vi "DataFinder_StorageVIs.vi"() -> ()   [LabVIEW 2023]
doc: "This example searches for channels in TDM files and TDMS files. The example uses the VIs \"Create Query\" and \"Execute Query\" to create and execute queries. The example then uses the \"Storage\" VIs to load the mass data of the found channels and graphically displays the data."
uses:
  <vilib>/DataFinder/DataTypes/object type.ctl
  <vilib>/DataFinder/DataTypes/comparison operator.ctl
  <vilib>/userdefined/High Color/DFDataFinder.ctl
  <vilib>/Platform/storage/lvStorage.llb/_openFunction.ctl
  <vilib>/DataFinder/Create Query (String).vi
  <vilib>/Platform/storage/lvStorage.llb/_openStorageWithRootAutoDetect.vi
  <vilib>/Platform/storage/lvStorage.llb/xStorage/xStorageSupp/ErrorOut.vi
  <vilib>/Platform/storage/lvStorage.llb/_queryPropPoly.vi
  <vilib>/Platform/storage/lvStorage.llb/_queryPropString.vi
  <vilib>/Platform/storage/lvStorage.llb/_queryGenericObjects.vi
  <vilib>/Platform/storage/lvStorage.llb/_loadAllDdt.vi
  <vilib>/Platform/storage/Storage.llb/Get Object Info.vi
  <vilib>/Platform/storage/Storage.llb/__closeStorageFromObject.vi
  <vilib>/DataFinder/Close Reference (Query).vi
  <vilib>/DataFinder/Close Reference (DataFinder).vi
  <vilib>/Platform/storage/lvStorage.llb/xStorage/Open Data Storage/Open Data Storage.xnode
  <vilib>/Platform/storage/lvStorage.llb/xStorage/Read Data/Read Data.xnode
  <vilib>/Platform/storage/lvStorage.llb/xStorage/Close Data Storage/Close Data Storage.xnode
  <vilib>/DataFinder/NI_DataFinder.lvlib
  <vilib>/userdefined/NI_DataFinder Controls.lvlib
panel:
  in  "DataFinder":T1
  in  "Operator":T2 items=["=", "<>", ">", "<", ">=", "<=", "#"]
  out "Result Signals":dynamicdata(graph)
  in  "Object Type":T3=2 items=["File", "Channel Group", "Channel"]
  in  "Value":string="Temp_A"
  in  "Property Name":string="name"
  out "Results Count":i32 min=0 max=0
  # "Overview: Executes a query for channels and uses the \"Storage\" VIs to display the mass data of the resulting channels.\nRequirements: Select a registered DataFinder which has indexed the TDM Server Demo Data.\nInstructions:\n1. Ensure that the selected DataFinder is already running.\n2. Specify a Query.\nTo use the predefined search values ensure the folder [all users]\\Documents\\National Instruments\\DataFinder or one of its parent folders is included in your search areas.\n3. Run the VI.\n4. View the Resulting Signals."
  # "Query"
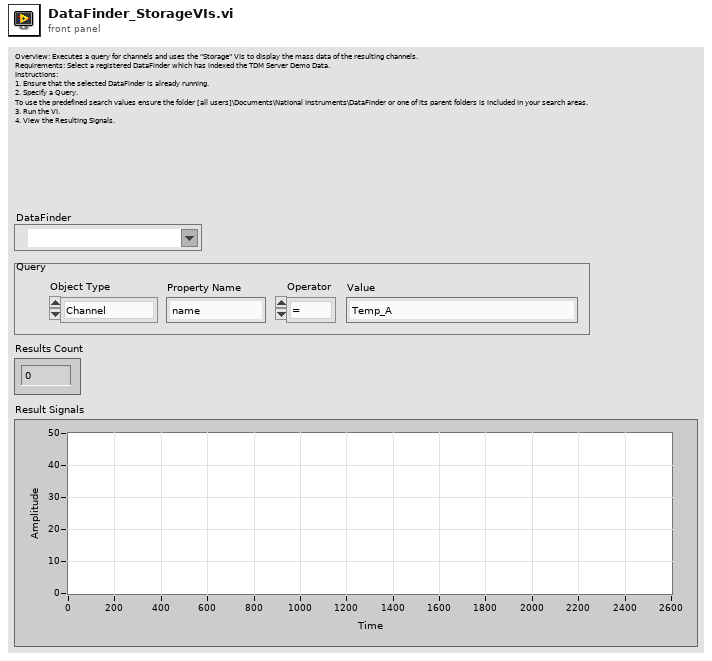
[diagram p1: front panel]
types:
  T1 = typedef "NI_DataFinder Controls.lvlib/DFDataFinder.ctl" = refnum<k21>
  T2 = typedef "NI_DataFinder.lvlib/comparison operator.ctl" = u16
  T3 = typedef "NI_DataFinder.lvlib/object type.ctl" = u16
  T4 = typedef "NI_DataFinder Controls.lvlib/DFQuery.ctl" = refnum<k20>
  T5 = typedef "NI_DataFinder.lvlib/results elements.ctl" = cluster{"fullpaths":path[], "DataPlugin names":string[], "channel group names":string[], "channel names":string[]}
  T6 = enum16{"UPDATE", "READ", "QUERY", "CREATE CHILD", "CREATE", "CONNECT", "DISCONNECT"}
  T7 = typedef "_openFunction.ctl" = enum16{"open", "open or create", "create or replace", "create", "open (read only)"}
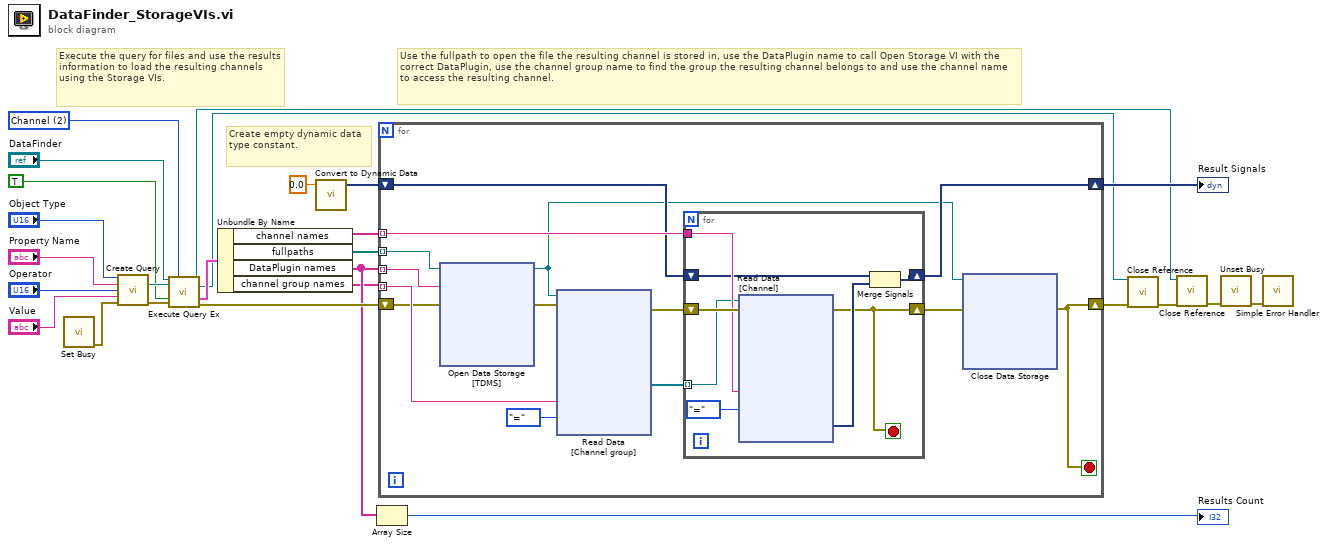
[diagram p0: block diagram]
diagram:
  w16 = T3 2 items=["File", "Channel Group", "Channel"] ("result object type (file)")
  # "Create empty dynamic data type constant."
  # "Use the fullpath to open the file the resulting channel is stored in, use the DataPlugin name to call Open Storage VI with the correct DataPlugin, use the channel group name to find the group the resulting channel belongs to and use the channel name to access the resulting channel."
  # "Execute the query for files and use the results information to load the resulting channels using the Storage VIs."
  n1 = call <vilib>:"Set Busy.vi"() -> ("error out"=w5:errorcluster)  [unwired: 10 in, 1 out]
  n2 = call-poly <vilib>:"Create Query.vi"("object type"="Object Type", "property name"="Property Name", "comparison operator (=)"="Operator", "value"="Value", "error in (no error)"=w5) -> ("query reference out"=w23:T4, "error out"=w24:errorcluster)  [unwired: 9 in]
  n3 = call <vilib>:"Execute Query Ex.vi"("DataFinder reference"="DataFinder", "result object type (file)"=w16, "query reference"=w23, "fill results elements? (F)"=TRUE, "error in (no error)"=w24) -> ("DataFinder reference out"=w9:T1, "query reference out"=w6:T4, "results elements"=w17:T5, "error out"=w18:errorcluster)  [unwired: 5 in, 2 out]
  n4 = Unbundle By Name(w17) -> ("channel names"=w12:string[], "fullpaths"=w13:path[], "DataPlugin names"=w15:string[], "channel group names"=w14:string[])
  n5 = call "Convert to Dynamic Data"("Double"=0.0) -> ("Dynamic Data Type"=w19:dynamicdata)  [unwired: 3 out]
  n6 = Array Size(array=w15) -> (size(s)=→"Results Count":i32)
  n7 = for {
    shift-right: [w33] -> w22
    shift-left: w19 -> [w34]
    shift-right: [w32] -> w8
    shift-left: w18 -> [w27]
    tunnel: w14 -> [w36] mode=indexing
    tunnel: w15 -> [w30] mode=indexing
    tunnel: w13 -> [w31] mode=indexing
    tunnel: w12 -> [w37] mode=indexing
    stop <- w32 stop-if-true
    n8 = xnode "Open Data Storage\n[TDMS]"("file path"=w31, "DataPlugin name"=w30, "error in (no error)"=w27) -> ("storage refnum (file)"=w28:refnum<k20>, "error out"=w29:errorcluster)  [unwired: 1 in, 2 out]
    n9 = xnode "Read Data\n[Channel group]"("Name"=w36, "Comparison (=)"=enum16{"=", "!=", ">", "<", ">=", "<="}."=", "storage refnum (file)"=w28, "error in"=w29) -> ("storage refnums (channel group)"=w35:refnum<k20>[], "error out"=w38:errorcluster)  [unwired: 1 out]
    n10 = for {
      tunnel: w37 -> [w71]
      shift-right: [w67] -> w33
      shift-left: w34 -> [w69]
      shift-right: [w65] -> w40
      shift-left: w38 -> [w72]
      tunnel: w35 -> [w66] mode=indexing
      stop <- w65 stop-if-true
      n11 = xnode "Read Data\n[Channel]"("Name"=w71, "Comparison (=)"=enum16{"=", "!=", ">", "<", ">=", "<="}."=", "storage refnum (channel group)"=w66, "error in"=w72) -> ("Signal"=w68:dynamicdata, "error out"=w65:errorcluster)  [unwired: 2 out]
      n12 = Merge Signals(w69, w68) -> (w67:dynamicdata)
    }
    n13 = xnode "Close Data Storage\n"("storage refnum (file)"=w28, "error in (no error)"=w40) -> ("error out"=w32:errorcluster)  [unwired: 1 out]
  }
  "Result Signals" <- w22
  n14 = call-poly <vilib>:"Close Reference.vi"("query reference"=w6, "error in (no error)"=w8) -> ("error out"=w7:errorcluster)  [unwired: 13 in]
  n15 = call-poly <vilib>:"Close Reference.vi"("DataFinder reference"=w9, "error in (no error)"=w7) -> ("error out"=w3:errorcluster)  [unwired: 13 in]
  n16 = call <vilib>:"Unset Busy.vi"("error in (no error)"=w3) -> ("error out"=w4:errorcluster)  [unwired: 10 in]
  n17 = call <vilib>:"Simple Error Handler.vi"("error in (no error)"=w4) -> ()  [unwired: 4 in, 5 out]
